vi "json_white.vi"(5 "text":string, 7 "ch":string, 9 "at":i32, 11 "error in (no error)":errorcluster) -> (6 "text dup":string, 8 "ch out":string, 10 "at out":i32, 15 "error out":errorcluster)   [LabVIEW 2011]
doc: "Skip white space until a non-whitespace character is found."
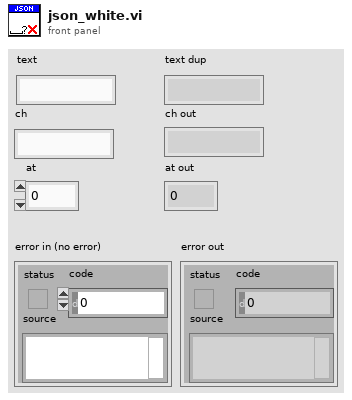
[diagram p1: front panel]
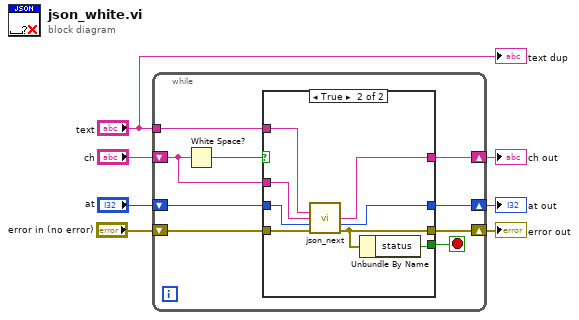
[diagram p0: block diagram]
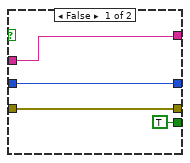
[diagram p2: hidden frame]
diagram:
  n1 = while {
    tunnel: "text" -> [w14]
    shift-right: [w13] -> w4
    shift-left: "at" -> [w15]
    shift-right: [w11] -> w3
    shift-left: "ch" -> [w10]
    shift-right: [w8] -> w1
    shift-left: "error in (no error)" -> [w9]
    stop <- w12 stop-if-true
    n2 = White Space?(1:w10) -> (0:w16:bool)
    n3 = case shown="True" w16 {
      tunnel: w15 -> [w20 w28]
      tunnel: w14 -> [_ w27]
      tunnel: [w20 w26] -> w13
      tunnel: [TRUE w21] -> w12
      tunnel: [w18 w25] -> w11
      tunnel: w10 -> [w18 w23]
      tunnel: w9 -> [w17 w24]
      tunnel: [w17 w22] -> w8
      frame False {
      }
      frame True {
        n4 = call "json_next.vi"("text"=w27, "ch"=w23, "at"=w28, "error in (no error)"=w24) -> ("ch out"=w25:string, "at out"=w26:i32, "error out"=w22:errorcluster)  [unwired: 8 in, 1 out]
        n5 = Unbundle By Name(w22) -> ("status"=w21:bool)
      }
    }
  }
  "at out" <- w4
  "ch out" <- w3
  "error out" <- w1
  "text dup" <- "text"
